vi "PH_PowerUnit_BaseClass.PC PU on.vi"(0 "i ref in":refnum<vi>, 2 "PU on":bool, 5 "error in (no error)":errorcluster) -> (14 "i ref out":refnum<vi>, 19 "error out":errorcluster)   [LabVIEW 2014, in "PH_PowerUnit_BaseClass.lvlib"]
doc: "This is the action VI of the PU on event case. Depending on the inout it does the following:\n\nfalse: set save state\ntrue: if the PreAmp is not disabled and State SM = \"Stand by\", a state change request is send to SM to get \"Switch PU on\" and the attribute \"PU in use\" is set to true. \nelse: GUI Knob is resetted"
uses:
  PH_PowerUnit_BaseClass.lvlib
  PH_Common/PH_Common.lvlib
  lib.lib/DimLVEvent/LVDimInterface/LVDimInterface.lvlib
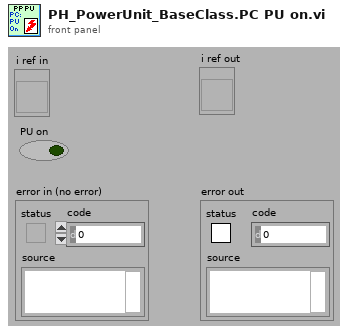
[diagram p1: front panel]
types:
  T1 = typedef "PH_PowerUnit_BaseClass.lvlib/PH_PowerUnit_BaseClass.i attribute.ctl" = cluster{"Constructor finished":bool, "PU":cluster{"In use":bool, "Service ID in use":i32, "GUI Ref":refnum<vi>}, "Enabling":cluster{"State":T2, "GUI Ref":refnum<vi>}, "Timing":cluster{"Last Shot":dbl, "Time between Shots [Sec]":dbl, "Waiting Time over?":bool, "Service ID Waiting Time":i32, "GUI Ref":refnum<vi>, "Instance":cluster{"Status":T3, "linked?":bool, "GUI Ref":refnum<vi>}}, "Sequencer":cluster{"SM State":string, "GUI Ref":refnum<vi>, "linked":bool}, "Subscribed Trendmssgs":cluster{"Tagname":string, "Status":T3, "linked?":bool, "Shot Condition":T3, "GUI Ref":refnum<vi>}[], "PP PU":T4, "Default Voltage (V)":dbl, "GUI Refs":T5, "PSDB data":cluster{"Shot Voltage [V]":dbl, "State TO SM":T6, "Write 2 early":bool}, "State TO SM":T6}
  T2 = typedef "PH_SystemInformation.lvlib/PH_SystemInformationEnabling State.ctl" = i32
  T3 = typedef "PH_StatusHandler.lvlib/PH_StatusHandler.Status.ctl" = i16
  T4 = typedef "PH_PP_Common.lvlib/PH_PP_Common.PUs.ctl" = enum16{"no Info", "PA-19mm-1", "PA-19mm-2", "PA-45mm-PILC", "PA-45mm-MAIN", "MA-PU-1", "MA-PU-2", "MA-PU-3", "MA-PU-4", "MA-PU-5", "MA-PU-6", "MA-FR", "MA-PILC", "PA-45mm-DP"}
  T5 = typedef "PH_PowerUnit_BaseClass.lvlib/PH_PowerUnit_BaseClass.GUI Refs.ctl" = cluster{"Delete Inst":refnum<vi>, "State TO SM":refnum<vi>, "State SM":refnum<vi>, "Fire":refnum<vi>}
  T6 = typedef "PH_PowerUnit_BaseClass.lvlib/PH_PowerUnit_BaseClass.SM States.ctl" = enum16{".", "Stand by", "Switch PU on", "Configure", "Set Default Voltage", "Set STANDBY", "Set READY", "Wait for Shot Cmd", "Open Dump Rods", "Open Ross Relais", "Close Ross Relais", "Switch PSU on", "Switch PSU off", "Charge", "Switch GD Channel on", "Close Dump Rods", "Rods-TO", "RR-TO", "PSU-TO", "Trigger-TO"}
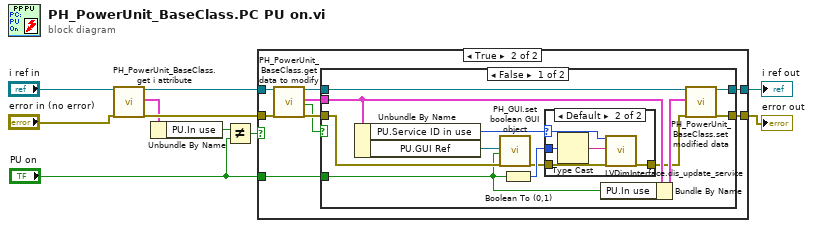
[diagram p0: block diagram]
diagram:
  n1 = call "PH_PowerUnit_BaseClass.get i attribute.vi"("i ref in"="i ref in", "error in (no error)"="error in (no error)") -> ("i ref out"=w6:refnum<vi>, "i attribute"=w4:T1, "error out"=w5:errorcluster)  [unwired: 15 in]
  n2 = Unbundle By Name(w4) -> ("PU.In use"=w3:bool)
  n3 = Not Equal?(x=w3, y="PU on") -> (x != y?=w1:bool)
  n4 = case shown="True" w1 {
    tunnel: [w12 w17] -> w10
    tunnel: [w11 w16] -> w9
    tunnel: w6 -> [w12 w15]
    tunnel: w5 -> [w11 w14]
    tunnel: "PU on" -> [_ w13]
    frame False {
    }
    frame True {
      n5 = call "PH_PowerUnit_BaseClass.get data to modify.vi"("i ref in"=w15, "error in (no error)"=w14) -> ("i ref out"=w19:refnum<vi>, "i attribute"=w21:T1, "timed out"=w18:bool, "error out"=w20:errorcluster)  [unwired: 14 in]
      n6 = case shown="False" w18 {
        tunnel: w13 -> [w26 _]
        tunnel: w21 -> [w29 _]
        tunnel: w20 -> [w27 w40]
        tunnel: w19 -> [w32 w41]
        tunnel: [w30 w41] -> w17
        tunnel: [w31 w40] -> w16
        frame False {
          n7 = Unbundle By Name(w29) -> ("PU.Service ID in use"=w24:i32, "PU.GUI Ref"=w28:refnum<vi>)
          n8 = call "PH_GUI.set boolean GUI object.vi"("Boolean Knob GUI Ref"=w28, "Value"=w26, "error in (no error)"=w27) -> ("error out"=w23:errorcluster)  [unwired: 16 in]
          n9 = Boolean To (0,1)(Boolean=w26) -> (0, 1=w25:i16)
          n10 = case shown="Default" w24 {
            selector: w24 -> [_ w37]
            tunnel: [w34 w38] -> w22
            tunnel: w23 -> [w34 w39]
            tunnel: w25 -> [_ w35]
            frame -1 {
            }
            frame Default {
              n11 = Type Cast(x=w35) -> (*(type *) &x=w36:string)  [unwired: 1 in]
              n12 = call "LVDimInterface.dis_update_service.vi"("my_serviceID"=w37, "data"=w36, "error in (no error)"=w39) -> ("error out"=w38:errorcluster)  [unwired: 14 in, 2 out]
            }
          }
          n13 = Bundle By Name(cluster=w29, "PU.In use"=w26) -> (w33:T1)
          n14 = call "PH_PowerUnit_BaseClass.set modified data.vi"("i ref in"=w32, "i attribute"=w33, "error in (no error)"=w22) -> ("i ref out"=w30:refnum<vi>, "error out"=w31:errorcluster)  [unwired: 15 in]
        }
        frame True {
        }
      }
    }
  }
  "error out" <- w9
  "i ref out" <- w10
